vi "ArmLiftControl.vi"(11 "Numeric":dbl) -> (2 "OnTarget":bool, 3 "OutputValue":dbl)   [LabVIEW 2020]
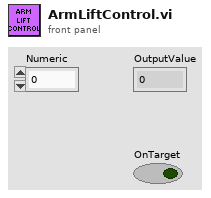
[diagram p1: front panel]
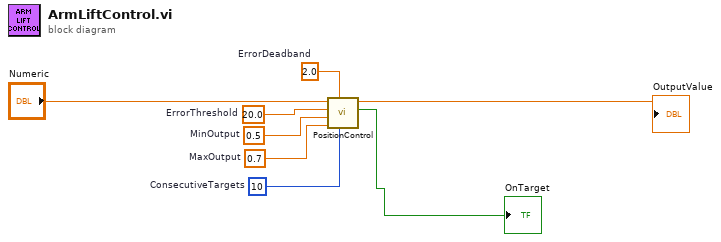
[diagram p0: block diagram]
diagram:
  w7 = 10  # ConsecutiveTargets
  w6 = 0.7  # MaxOutput
  w5 = 0.5  # MinOutput
  w4 = 20.0  # ErrorThreshold
  w2 = 2.0  # ErrorDeadband
  n1 = call "PositionControl.vi"("ConsecutiveTargets"=w7, "ErrorDeadband"=w2, "MaxOutput"=w6, "MinOutput"=w5, "ErrorThreshold"=w4, "Error"="Numeric") -> ("OnTarget"=→"OnTarget":bool, "OutputValue"=→"OutputValue":dbl)  [unwired: 3 in, 1 out]
